vi "mainAuto.vi"() -> ()   [LabVIEW 2018]
uses:
  MotorController/#include/Global textParse.vi
panel:
  in  "Device Type":bool caption="Boolean"
  in  "Number of Oscilloscopes":bool caption="Boolean"
  in  "SpecSheet Scan":string
  in  "PO Line#":string
  in  "PO#":string
  in  "Number":string
  in  "Vendor":string
  in  "Station":string
  in  "Inspector":string
  in  "Inspection Point":string(combo)
  in  "VISA Oscilloscope 2":refnum<visa-resource-name>
  in  "VISA Oscilloscope 1":refnum<visa-resource-name>
  in  "Serial Port":refnum<visa-resource-name>
  in  "E-Stop":bool
  out "Initialize":string
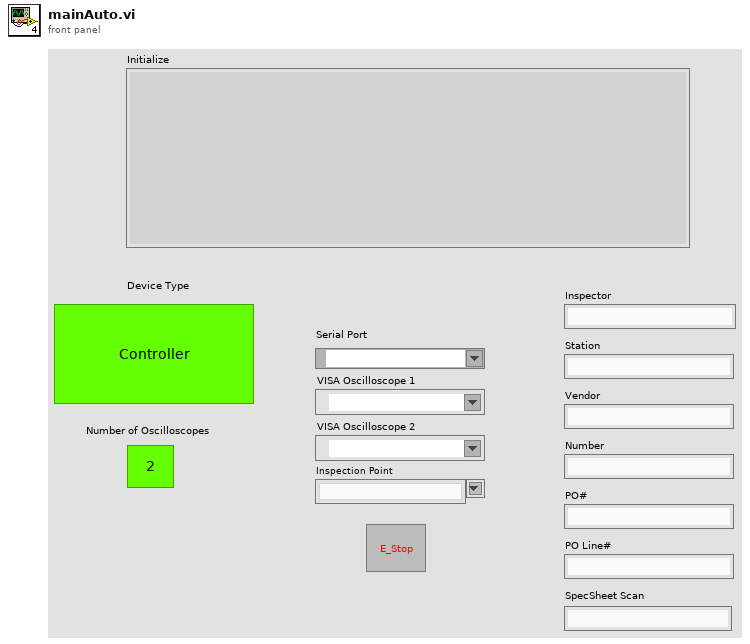
[diagram p1: front panel]
types:
  T1 = enum16{"initialize", "test", "pass/fail", "finish"}
  T2 = enum16{"Scan/Read", "Secondary", "Incline", "Motor"}
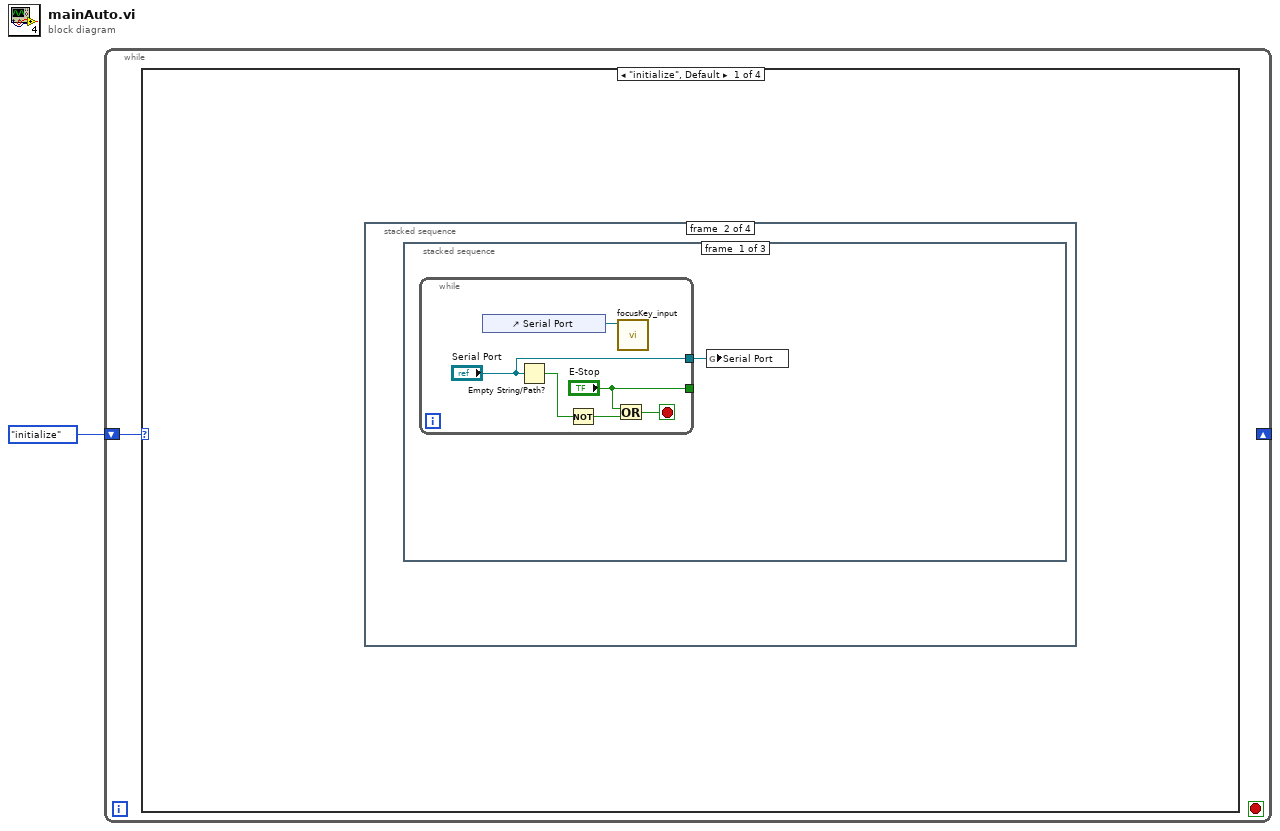
[diagram p0: block diagram]
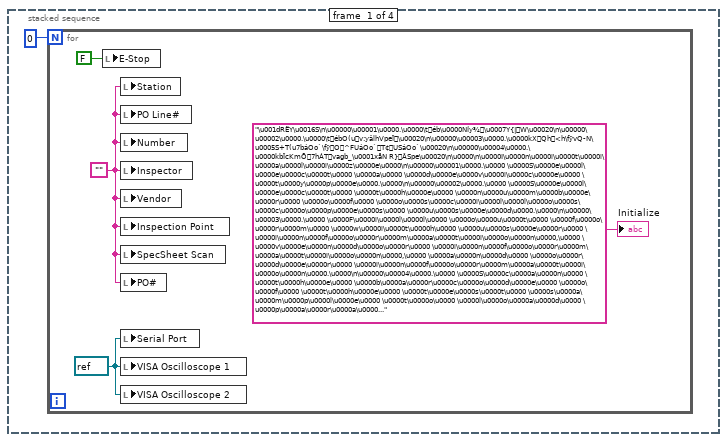
[diagram p2: hidden frame]
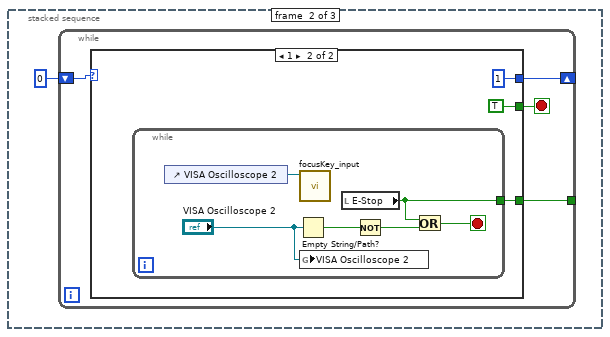
[diagram p3: hidden frame]
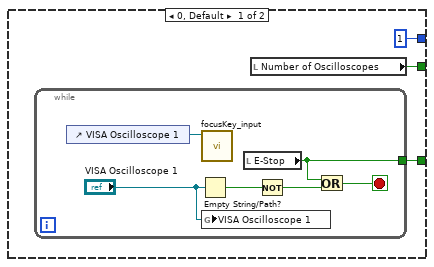
[diagram p4: hidden frame]
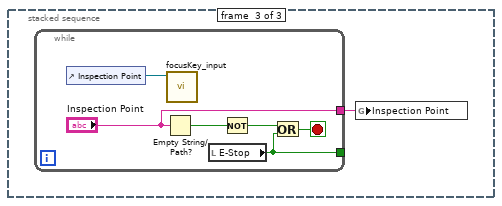
[diagram p5: hidden frame]
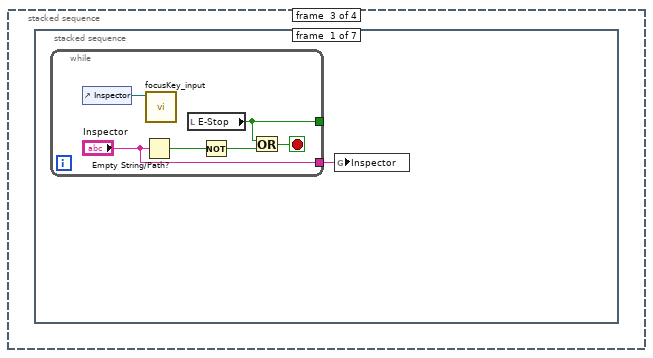
[diagram p6: hidden frame]
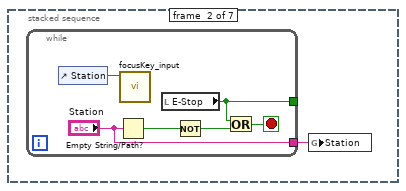
[diagram p7: hidden frame]
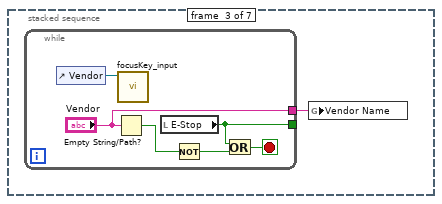
[diagram p8: hidden frame]
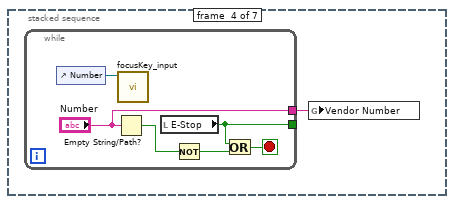
[diagram p9: hidden frame]
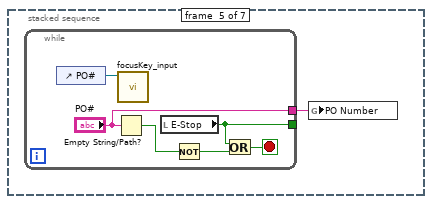
[diagram p10: hidden frame]
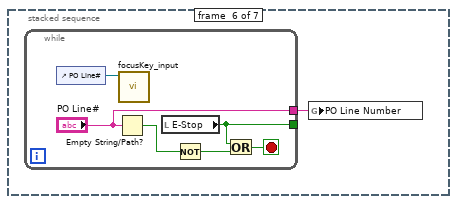
[diagram p11: hidden frame]
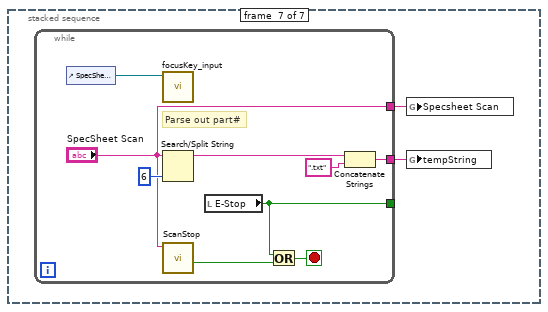
[diagram p12: hidden frame]
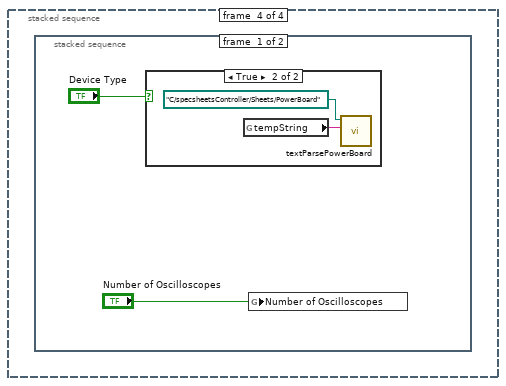
[diagram p13: hidden frame]
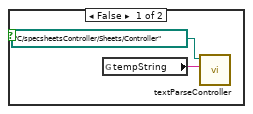
[diagram p14: hidden frame]
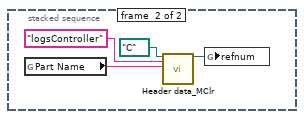
[diagram p15: hidden frame]
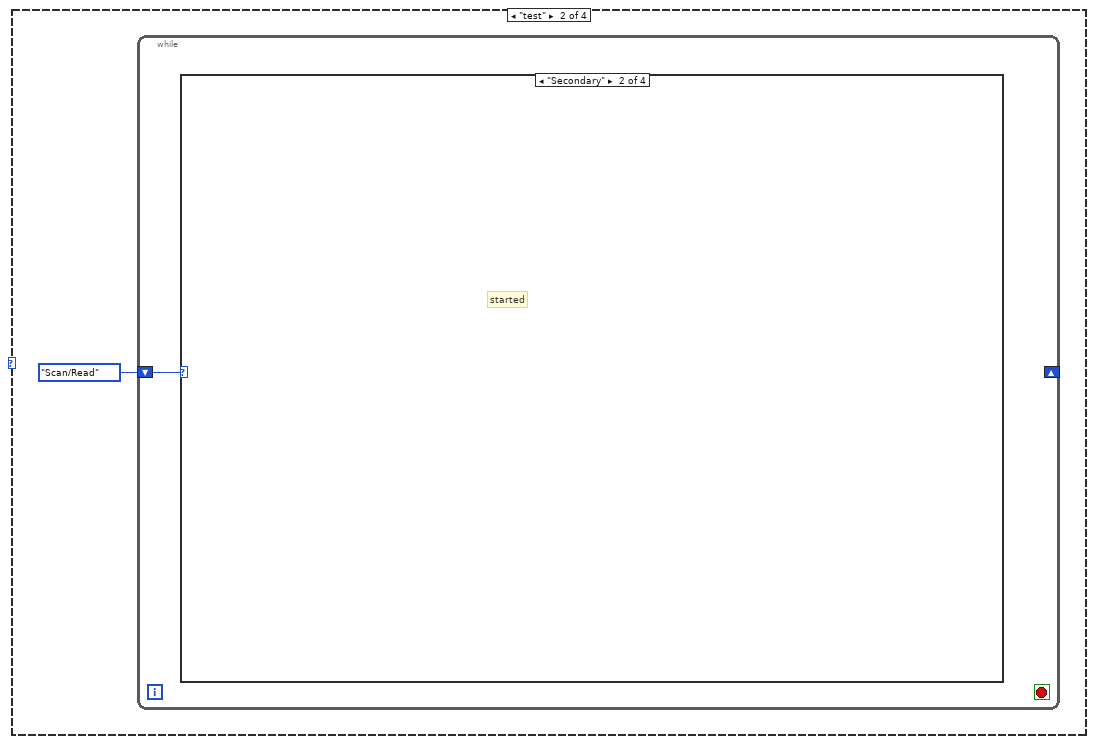
[diagram p16: hidden frame]
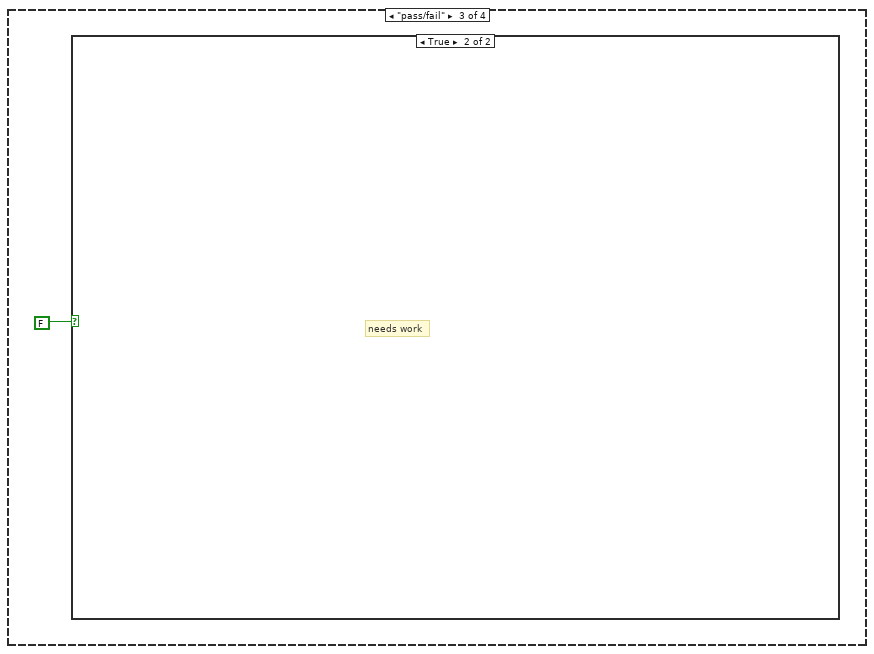
[diagram p20: hidden frame]
diagram:
  n1 = while {
    shift-right: _ -> [_]
    shift-left: T1."initialize" -> [w2]
    stop <- _ stop-if-true
    n2 = case shown="\"initialize\", Default" w2 {
      frame "initialize", Default {
        n3 = stacked-sequence {
          frame #0 {
            n4 = for {
              N: 0 -> [_]
              w5 = ""
              w6 = refnum<visa-resource-name> refnum ("VISA Oscilloscope 1")
              n5 = local write "E-Stop"(FALSE ("E-Stop")) -> ()
              n6 = local write "Station"(w5) -> ()
              n7 = local write "PO Line#"(w5) -> ()
              n8 = local write "Number"(w5) -> ()
              n9 = local write "Inspector"(w5) -> ()
              n10 = local write "Vendor"(w5) -> ()
              n11 = local write "Inspection Point"(w5) -> ()
              n12 = local write "SpecSheet Scan"(w5) -> ()
              n13 = local write "PO#"(w5) -> ()
              n14 = local write "Serial Port"(w6) -> ()
              n15 = local write "VISA Oscilloscope 1"(w6) -> ()
              n16 = local write "VISA Oscilloscope 2"(w6) -> ()
              "Initialize" <- "\u001dRËY\u0016S\n\u00000\u00001\u0000.\u0000\téb\u0000NÍy¾\u0007Y{|W\u00020\n\u00000\u00002\u0000.\u0000\tébO(uv:yâlhVpeÏ\u00020\n\u00000\u00003\u0000.\u0000kXQh<h\fÿvQ-N\u0005S+T(u7báOo`\fÿO^FUáOo`T¢USáOo`\u00020\n\u00000\u00004\u0000.\u0000kbÏcKmÕ7hÁTvagb_\u0001xåN R}ÂSpe\u00020\n\u0000\n\u0000I\u0000n\u0000i\u0000t\u0000i\u0000a\u0000l\u0000i\u0000z\u0000e\u0000\n\u00000\u00001\u0000.\u0000 \u0000S\u0000e\u0000l\u0000e\u0000c\u0000t\u0000 \u0000a\u0000 \u0000d\u0000e\u0000v\u0000i\u0000c\u0000e\u0000 \u0000t\u0000y\u0000p\u0000e\u0000.\u0000\n\u00000\u00002\u0000.\u0000 \u0000S\u0000e\u0000l\u0000e\u0000c\u0000t\u0000 \u0000t\u0000h\u0000e\u0000 \u0000n\u0000u\u0000m\u0000b\u0000e\u0000r\u0000 \u0000o\u0000f\u0000 \u0000o\u0000s\u0000c\u0000i\u0000l\u0000l\u0000o\u0000s\u0000c\u0000o\u0000p\u0000e\u0000s\u0000 \u0000u\u0000s\u0000e\u0000d\u0000.\u0000\n\u00000\u00003\u0000.\u0000 \u0000F\u0000i\u0000l\u0000l\u0000 \u0000o\u0000u\u0000t\u0000 \u0000f\u0000o\u0000r\u0000m\u0000 \u0000w\u0000i\u0000t\u0000h\u0000 \u0000u\u0000s\u0000e\u0000r\u0000 \u0000i\u0000n\u0000f\u0000o\u0000r\u0000m\u0000a\u0000t\u0000i\u0000o\u0000n\u0000,\u0000 \u0000v\u0000e\u0000n\u0000d\u0000o\u0000r\u0000 \u0000i\u0000n\u0000f\u0000o\u0000r\u0000m\u0000a\u0000t\u0000i\u0000o\u0000n\u0000,\u0000 \u0000a\u0000n\u0000d\u0000 \u0000o\u0000r\u0000d\u0000e\u0000r\u0000 \u0000i\u0000n\u0000f\u0000o\u0000r\u0000m\u0000a\u0000t\u0000i\u0000o\u0000n\u0000.\u0000\n\u00000\u00004\u0000.\u0000 \u0000S\u0000c\u0000a\u0000n\u0000 \u0000t\u0000h\u0000e\u0000 \u0000b\u0000a\u0000r\u0000c\u0000o\u0000d\u0000e\u0000 \u0000o\u0000f\u0000 \u0000t\u0000h\u0000e\u0000 \u0000t\u0000e\u0000s\u0000t\u0000 \u0000s\u0000a\u0000m\u0000p\u0000l\u0000e\u0000 \u0000t\u0000o\u0000 \u0000l\u0000o\u0000a\u0000d\u0000 \u0000p\u0000a\u0000r\u0000a\u0000..."
            }
          }
          frame #1 {
            n17 = stacked-sequence {
              frame #0 {
                n18 = while {
                  tunnel: ["E-Stop"] -> _
                  tunnel: ["Serial Port"] -> w8
                  stop <- w11 stop-if-true
                  n19 = control-ref of="Serial Port"() -> (w13:refnum<vi>)
                  n20 = Empty String/Path?(string/path="Serial Port") -> (empty?=w14:bool)
                  n21 = Not(x=w14) -> (.not. x?=w12:bool)
                  n22 = Or(x="E-Stop", y=w12) -> (x .or. y?=w11:bool)
                  n23 = call "focusKey_input.vi"("reference"=w13) -> ()  [unwired: 10 in, 1 out]
                }
                n24 = global write "Global textParse.vi" "Serial Port"(w8) -> ()
              }
              frame #1 {
                n25 = while {
                  shift-right: [w16] -> _
                  shift-left: 0 -> [w19]
                  tunnel: [w18] -> _
                  stop <- w17 stop-if-true
                  n26 = case shown="1" w19 {
                    tunnel: [w20 w31] -> w18
                    tunnel: [w22 TRUE] -> w17
                    tunnel: [1 1] -> w16
                    frame 0, Default {
                      n27 = while {
                        tunnel: [w24] -> w20
                        stop <- w26 stop-if-true
                        n28 = control-ref of="VISA Oscilloscope 1"() -> (w27:refnum<vi>)
                        n29 = Empty String/Path?(string/path="VISA Oscilloscope 1") -> (empty?=w28:bool)
                        n30 = call "focusKey_input.vi"("reference"=w27) -> ()  [unwired: 10 in, 1 out]
                        n31 = global write "Global textParse.vi" "VISA Oscilloscope 1"("VISA Oscilloscope 1") -> ()
                        n32 = local read "E-Stop"() -> (w24:bool)
                        n33 = Not(x=w28) -> (.not. x?=w25:bool)
                        n34 = Or(x=w24, y=w25) -> (x .or. y?=w26:bool)
                      }
                      n35 = local read "Number of Oscilloscopes"() -> (w22:bool)
                    }
                    frame 1 {
                      n36 = while {
                        tunnel: [w33] -> w31
                        stop <- w35 stop-if-true
                        n37 = control-ref of="VISA Oscilloscope 2"() -> (w36:refnum<vi>)
                        n38 = Empty String/Path?(string/path="VISA Oscilloscope 2") -> (empty?=w37:bool)
                        n39 = call "focusKey_input.vi"("reference"=w36) -> ()  [unwired: 10 in, 1 out]
                        n40 = global write "Global textParse.vi" "VISA Oscilloscope 2"("VISA Oscilloscope 2") -> ()
                        n41 = local read "E-Stop"() -> (w33:bool)
                        n42 = Not(x=w37) -> (.not. x?=w34:bool)
                        n43 = Or(x=w33, y=w34) -> (x .or. y?=w35:bool)
                      }
                    }
                  }
                }
              }
              frame #2 {
                n44 = while {
                  tunnel: [w40] -> _
                  tunnel: ["Inspection Point"] -> w38
                  stop <- w44 stop-if-true
                  n45 = control-ref of="Inspection Point"() -> (w41:refnum<vi>)
                  n46 = Empty String/Path?(string/path="Inspection Point") -> (empty?=w43:bool)
                  n47 = call "focusKey_input.vi"("reference"=w41) -> ()  [unwired: 10 in, 1 out]
                  n48 = local read "E-Stop"() -> (w40:bool)
                  n49 = Not(x=w43) -> (.not. x?=w42:bool)
                  n50 = Or(x=w42, y=w40) -> (x .or. y?=w44:bool)
                }
                n51 = global write "Global textParse.vi" "Inspection Point"(w38) -> ()
              }
            }
          }
          frame #2 {
            n52 = stacked-sequence {
              frame #0 {
                n53 = while {
                  tunnel: ["Inspector"] -> w45
                  tunnel: [w46] -> _
                  stop <- w48 stop-if-true
                  n54 = control-ref of="Inspector"() -> (w49:refnum<vi>)
                  n55 = Empty String/Path?(string/path="Inspector") -> (empty?=w51:bool)
                  n56 = call "focusKey_input.vi"("reference"=w49) -> ()  [unwired: 10 in, 1 out]
                  n57 = local read "E-Stop"() -> (w46:bool)
                  n58 = Not(x=w51) -> (.not. x?=w47:bool)
                  n59 = Or(x=w46, y=w47) -> (x .or. y?=w48:bool)
                }
                n60 = global write "Global textParse.vi" "Inspector"(w45) -> ()
              }
              frame #1 {
                n61 = while {
                  tunnel: ["Station"] -> w52
                  tunnel: [w53] -> _
                  stop <- w55 stop-if-true
                  n62 = control-ref of="Station"() -> (w56:refnum<vi>)
                  n63 = Empty String/Path?(string/path="Station") -> (empty?=w58:bool)
                  n64 = call "focusKey_input.vi"("reference"=w56) -> ()  [unwired: 10 in, 1 out]
                  n65 = local read "E-Stop"() -> (w53:bool)
                  n66 = Not(x=w58) -> (.not. x?=w54:bool)
                  n67 = Or(x=w53, y=w54) -> (x .or. y?=w55:bool)
                }
                n68 = global write "Global textParse.vi" "Station"(w52) -> ()
              }
              frame #2 {
                n69 = while {
                  tunnel: ["Vendor"] -> w59
                  tunnel: [w60] -> _
                  stop <- w62 stop-if-true
                  n70 = control-ref of="Vendor"() -> (w63:refnum<vi>)
                  n71 = Empty String/Path?(string/path="Vendor") -> (empty?=w65:bool)
                  n72 = call "focusKey_input.vi"("reference"=w63) -> ()  [unwired: 10 in, 1 out]
                  n73 = local read "E-Stop"() -> (w60:bool)
                  n74 = Not(x=w65) -> (.not. x?=w61:bool)
                  n75 = Or(x=w60, y=w61) -> (x .or. y?=w62:bool)
                }
                n76 = global write "Global textParse.vi" "Vendor Name"(w59) -> ()
              }
              frame #3 {
                n77 = while {
                  tunnel: ["Number"] -> w66
                  tunnel: [w67] -> _
                  stop <- w69 stop-if-true
                  n78 = control-ref of="Number"() -> (w70:refnum<vi>)
                  n79 = Empty String/Path?(string/path="Number") -> (empty?=w72:bool)
                  n80 = call "focusKey_input.vi"("reference"=w70) -> ()  [unwired: 10 in, 1 out]
                  n81 = local read "E-Stop"() -> (w67:bool)
                  n82 = Not(x=w72) -> (.not. x?=w68:bool)
                  n83 = Or(x=w67, y=w68) -> (x .or. y?=w69:bool)
                }
                n84 = global write "Global textParse.vi" "Vendor Number"(w66) -> ()
              }
              frame #4 {
                n85 = while {
                  tunnel: ["PO#"] -> w73
                  tunnel: [w74] -> _
                  stop <- w76 stop-if-true
                  n86 = control-ref of="PO#"() -> (w77:refnum<vi>)
                  n87 = Empty String/Path?(string/path="PO#") -> (empty?=w79:bool)
                  n88 = call "focusKey_input.vi"("reference"=w77) -> ()  [unwired: 10 in, 1 out]
                  n89 = local read "E-Stop"() -> (w74:bool)
                  n90 = Not(x=w79) -> (.not. x?=w75:bool)
                  n91 = Or(x=w74, y=w75) -> (x .or. y?=w76:bool)
                }
                n92 = global write "Global textParse.vi" "PO Number"(w73) -> ()
              }
              frame #5 {
                n93 = while {
                  tunnel: ["PO Line#"] -> w80
                  tunnel: [w81] -> _
                  stop <- w85 stop-if-true
                  n94 = control-ref of="PO Line#"() -> (w83:refnum<vi>)
                  n95 = Empty String/Path?(string/path="PO Line#") -> (empty?=w84:bool)
                  n96 = call "focusKey_input.vi"("reference"=w83) -> ()  [unwired: 10 in, 1 out]
                  n97 = local read "E-Stop"() -> (w81:bool)
                  n98 = Not(x=w84) -> (.not. x?=w86:bool)
                  n99 = Or(x=w81, y=w86) -> (x .or. y?=w85:bool)
                }
                n100 = global write "Global textParse.vi" "PO Line Number"(w80) -> ()
              }
              frame #6 {
                n101 = while {
                  tunnel: ["SpecSheet Scan"] -> w88
                  tunnel: [w93] -> w87
                  tunnel: [w89] -> _
                  stop <- w90 stop-if-true
                  # "Parse out part#"
                  n102 = control-ref of="SpecSheet Scan"() -> (w97:refnum<vi>)
                  n103 = call "focusKey_input.vi"("reference"=w97) -> ()  [unwired: 10 in, 1 out]
                  n104 = Search/Split String(string="SpecSheet Scan", offset (0)=6) -> (substring before match=w94:string)  [unwired: 1 in, 2 out]
                  n105 = call "ScanStop.vi"("bar code scan"="SpecSheet Scan") -> ("Output"=w92:bool)  [unwired: 8 in, 2 out]
                  n106 = local read "E-Stop"() -> (w89:bool)
                  n107 = Or(x=w89, y=w92) -> (x .or. y?=w90:bool)
                  n108 = Concatenate Strings(w94, ".txt" ("string")) -> (w93:string)
                }
                n109 = global write "Global textParse.vi" "Specsheet Scan"(w88) -> ()
                n110 = global write "Global textParse.vi" "tempString"(w87) -> ()
              }
            }
          }
          frame #3 {
            n111 = stacked-sequence {
              frame #0 {
                n112 = case shown="True" "Device Type" {
                  frame False {
                    n113 = global read "Global textParse.vi" "tempString"() -> (w101:string)
                    n114 = call "textParseController.vi"("file name"=w101, "base path"=path "C:/specsheetsController/Sheets/Controller") -> ()  [unwired: 7 in, 3 out]
                  }
                  frame True {
                    n115 = global read "Global textParse.vi" "tempString"() -> (w103:string)
                    n116 = call "textParsePowerBoard.vi"("file name"=w103, "base path"=path "C:/specsheetsController/Sheets/PowerBoard") -> ()  [unwired: 7 in, 3 out]
                  }
                }
                n117 = global write "Global textParse.vi" "Number of Oscilloscopes"("Number of Oscilloscopes") -> ()
              }
              frame #1 {
                n118 = global read "Global textParse.vi" "Part Name"() -> (w107:string)
                n119 = call "Header data_MClr.vi"("base path"=path "C:/", "prompt (Create Folder)"="logsController", "file name"=w107) -> ("refnum out"=w104:refnum<file>)  [unwired: 15 in, 1 out]
                n120 = global write "Global textParse.vi" "refnum"(w104) -> ()
              }
            }
          }
        }
      }
      frame "test" {
        n121 = while {
          shift-right: _ -> [_]
          shift-left: T2."Scan/Read" -> [w109]
          stop <- _ stop-if-true
          n122 = case shown="\"Secondary\"" w109 {
            frame "Scan/Read", Default {
              # "about done"
            }
            frame "Secondary" {
              # "started"
            }
            frame "Incline" {
              # "needs work"
            }
            frame "Motor" {
              # "needs work"
            }
          }
        }
      }
      frame "pass/fail" {
        n123 = case shown="True" FALSE {
          frame False {
          }
          frame True {
            # "needs work"
          }
        }
      }
      frame "finish" {
        n124 = flat-sequence {
          frame #0 {
            # "needs work"
          }
        }
      }
    }
  }
